vi "FestoCPX.DO.Data.States.Reset.vi"(6 "Timeout [ms] (0)":u32, 8 "error in (no error)":errorcluster) -> (0 "error out":errorcluster)   [LabVIEW 2016]
uses:
  FestoCPX.DO.Data.Fglb.Action.ctl
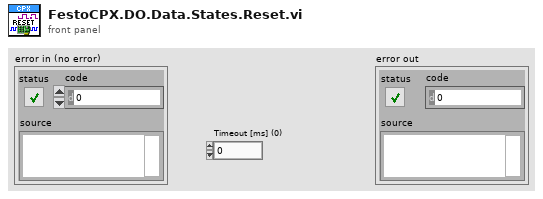
[diagram p1: front panel]
types:
  T1 = typedef "FestoCPX.DO.Data.Fglb.Action.ctl" = enum16{"init", "set", "get", "check", "select", "reset"}
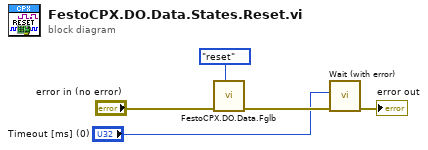
[diagram p0: block diagram]
diagram:
  n1 = call "FestoCPX.DO.Data.Fglb.vi"("state (get all)"=FestoCPX.DO.Data.Fglb.Action."reset", "error in (no error)"="error in (no error)") -> ("error out"=w3:errorcluster)  [unwired: 7 in, 2 out]
  n2 = call "Wait (with error).vi"("error in (no error)"=w3, "milliseconds to wait"="Timeout [ms] (0)") -> ("error out"=→"error out":errorcluster)  [unwired: 8 in, 1 out]
